vi "test_Import Bitfile Scalars_Label_Error.vi"(8 "error in (no error)":errorcluster, 11 "TestCase in":refnum<class "FPGA Addon Scripting API Unit Tests.lvclass">) -> (0 "error out":errorcluster, 3 "TestCase out":refnum<class "FPGA Addon Scripting API Unit Tests.lvclass">)   [LabVIEW 2021, in "FPGA Addon Scripting API Unit Tests.lvclass"]
uses:
  FPGA Addon Scripting API Unit Tests.lvclass
  APIs/Scripting API/TypeDefs/Input Scalar Data.ctl
  APIs/Scripting API/Public/Bitfile Resources/Import Bitfile Scalars (Instances)/Import Scalars - by label.vi
  <vilib>/addons/_JKI Toolkits/VI Tester/TestCase.llb/TestCase.lvclass
  FPGA Addon Test Class/FPGA Addon Test Class.lvclass
  APIs/Scripting API/Scripting API.lvlib
  C:/Program Files/National Instruments/LabVIEW 2021/vi.lib/addons/_JKI Toolkits/VI Tester/TestCase.llb/TestCase.lvclass
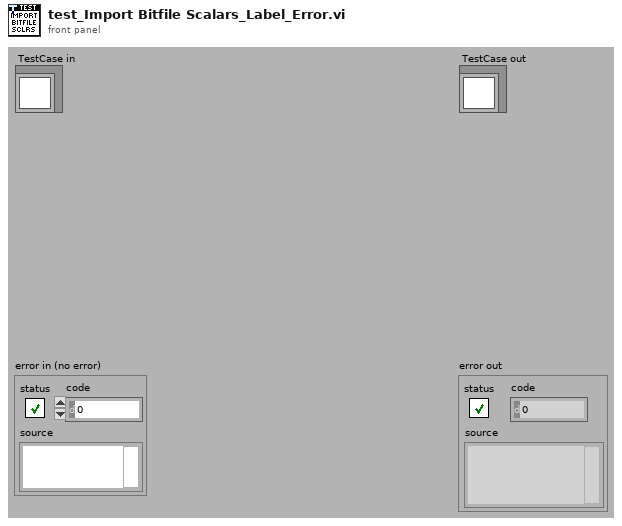
[diagram p1: front panel]
types:
  T1 = typedef "Scripting API.lvlib/Input Scalar Data.ctl" = cluster{"Bitfile Name":string, "SysDef Name":string}
  T2 = typedef "Custom Device API.lvlib/Custom Device Item Ref.ctl" = u64
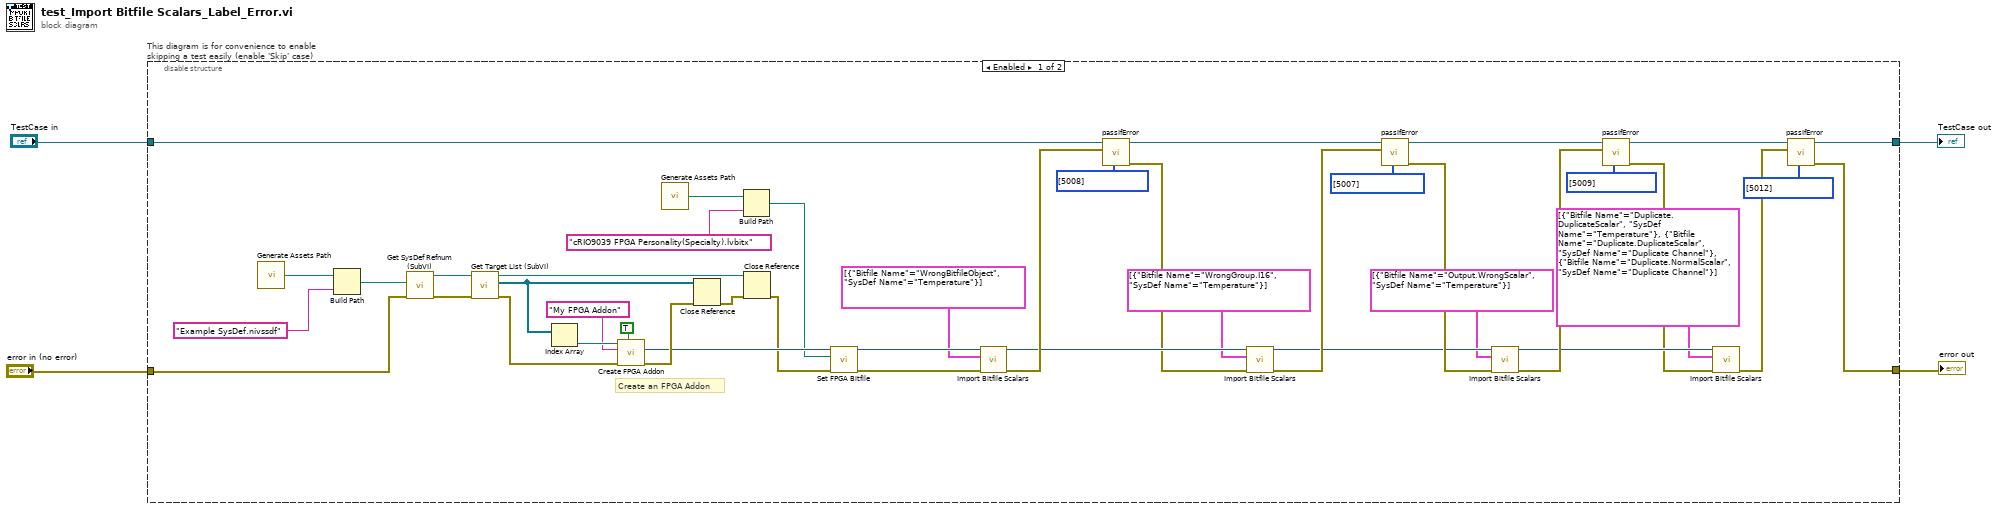
[diagram p0: block diagram]
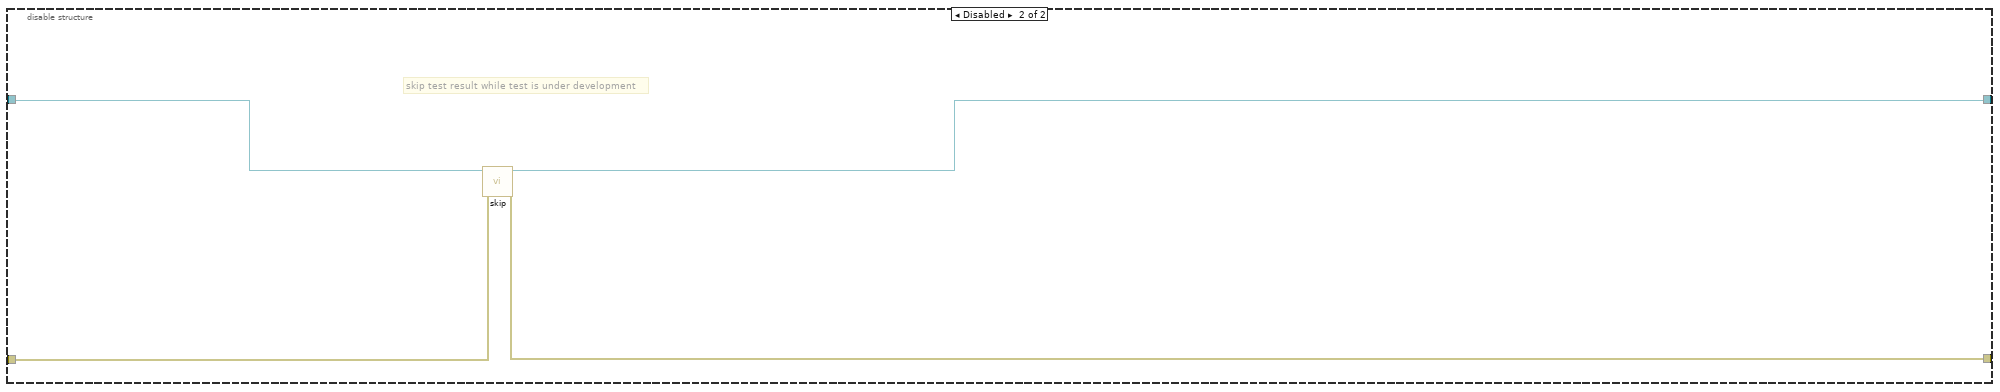
[diagram p2: hidden frame]
diagram:
  n1 = disable-structure "This diagram is for convenience to enable skipping a test easily (enable 'Skip' case)" shown="Enabled" {
    disable-tunnel: "TestCase in" -> [w27 w53]
    disable-tunnel: [w5 w51] -> w1
    disable-tunnel: [w6 w52] -> w3
    disable-tunnel: "error in (no error)" -> [w43 w50]
    frame Enabled {
      # "Create an FPGA Addon"
      n2 = call "Generate Assets Path.vi"() -> ("Assets path"=w49:path)
      n3 = Build Path(base path=w49, name or relative path="Example SysDef.nivssdf") -> (appended path=w47:path)
      n4 = call "Get SysDef Refnum (SubVI).vi"("error in (no error)"=w43, "System Definition path"=w47) -> ("error out"=w42:errorcluster, "SysDef Refnum out"=w46:refnum<k24>)  [unwired: 8 in]
      n5 = call "Get Target List (SubVI).vi"("error in (no error)"=w42, "SysDef Refnum in"=w46) -> ("error out"=w41:errorcluster, "Target List Refnums"=w40:refnum<k24>[], "SysDef Refnum out"=w39:refnum<k24>)  [unwired: 7 in]
      n6 = Index Array(array=w40) -> (element=w45:refnum<k24>)  [unwired: 1 in]
      n7 = call "Create FPGA Addon.vi"("group scalars"=TRUE, "error in"=w41, "FPGA addon name"="My FPGA Addon", "target in"=w45) -> ("error out"=w37:errorcluster, "FPGA addon refnum"=w35:T2)  [unwired: 5 in, 1 out]
      n8 = call "Generate Assets Path.vi"() -> ("Assets path"=w33:path)
      n9 = Close Reference(reference=w40, error in (no error)=w37) -> (error out=w38:errorcluster)
      n10 = Build Path(base path=w33, name or relative path="cRIO9039 FPGA Personality(Specialty).lvbitx") -> (appended path=w31:path)
      n11 = Close Reference(reference=w39, error in (no error)=w38) -> (error out=w34:errorcluster)
      n12 = call "Set FPGA Bitfile.vi"("error in"=w34, "FPGA bitfile path"=w31, "FPGA addon refnum in"=w35) -> ("error out"=w30:errorcluster, "FPGA addon refnum out"=w29:T2)  [unwired: 7 in]
      n13 = call-poly "Import Bitfile Scalars.vi"("error in"=w30, "bitfile scalars in"=T1[] [{"Bitfile Name"="WrongBitfileObject", "SysDef Name"="Temperature"}], "FPGA addon refnum in"=w29) -> ("error out"=w26:errorcluster, "FPGA addon refnum out"=w24:T2)  [unwired: 6 in, 1 out]
      n14 = call-dynamic "passIfError.vi"("passing error codes (default = any error code)"=i32[] [5008], "error"=w26, "TestCase in"=w27) -> ("error out"=w23:errorcluster, "TestCase out"=w21:refnum<class "FPGA Addon Scripting API Unit Tests.lvclass">)  [unwired: 7 in]
      n15 = call-poly "Import Bitfile Scalars.vi"("error in"=w23, "bitfile scalars in"=T1[] [{"Bitfile Name"="WrongGroup.I16", "SysDef Name"="Temperature"}], "FPGA addon refnum in"=w24) -> ("error out"=w20:errorcluster, "FPGA addon refnum out"=w17:T2)  [unwired: 6 in, 1 out]
      n16 = call-dynamic "passIfError.vi"("passing error codes (default = any error code)"=i32[] [5007], "error"=w20, "TestCase in"=w21) -> ("error out"=w18:errorcluster, "TestCase out"=w15:refnum<class "FPGA Addon Scripting API Unit Tests.lvclass">)  [unwired: 7 in]
      n17 = call-poly "Import Bitfile Scalars.vi"("error in"=w18, "bitfile scalars in"=T1[] [{"Bitfile Name"="Output.WrongScalar", "SysDef Name"="Temperature"}], "FPGA addon refnum in"=w17) -> ("error out"=w14:errorcluster, "FPGA addon refnum out"=w12:T2)  [unwired: 6 in, 1 out]
      n18 = call-dynamic "passIfError.vi"("passing error codes (default = any error code)"=i32[] [5009], "error"=w14, "TestCase in"=w15) -> ("error out"=w11:errorcluster, "TestCase out"=w9:refnum<class "FPGA Addon Scripting API Unit Tests.lvclass">)  [unwired: 7 in]
      n19 = call-poly "Import Bitfile Scalars.vi"("error in"=w11, "bitfile scalars in"=T1[] [{"Bitfile Name"="Duplicate.DuplicateScalar", "SysDef Name"="Temperature"}, {"Bitfile Name"="Duplicate.DuplicateScalar", "SysDef Name"="Duplicate Channel"}, {"Bitfile Name"="Duplicate.NormalScalar", "SysDef Name"="Duplicate Channel"}], "FPGA addon refnum in"=w12) -> ("error out"=w8:errorcluster)  [unwired: 6 in, 2 out]
      n20 = call-dynamic "passIfError.vi"("passing error codes (default = any error code)"=i32[] [5012], "error"=w8, "TestCase in"=w9) -> ("error out"=w6:errorcluster, "TestCase out"=w5:refnum<class "FPGA Addon Scripting API Unit Tests.lvclass">)  [unwired: 7 in]
    }
    frame Disabled {
      # "skip test result while test is under development"
      n21 = call <vilib>:"skip.vi"("error in (no error)"=w50, "TestCase in"=w53) -> ("error out"=w52:errorcluster, "TestCase out"=w51:refnum<class "FPGA Addon Scripting API Unit Tests.lvclass">)  [unwired: 8 in]
    }
  }
  "error out" <- w3
  "TestCase out" <- w1
